vi "Get Item Data.vi"(8 "error in (no error)":errorcluster, 11 "VI":refnum<vi>) -> (0 "error out":errorcluster, 2 "VI Data":T1, 3 "VI out":refnum<vi>)   [LabVIEW 2023, in "VI Properties Editor.lvlib"]
doc: "Gets all item data from the <B>VI</B>."
uses:
  VI Properties Editor.lvlib
  <vilib>/picture/picture.llb/imagedata.ctl
  CTLs/VI Data.ctl
  CTLs/Control Properties.ctl
  CTLs/VI Properties.ctl
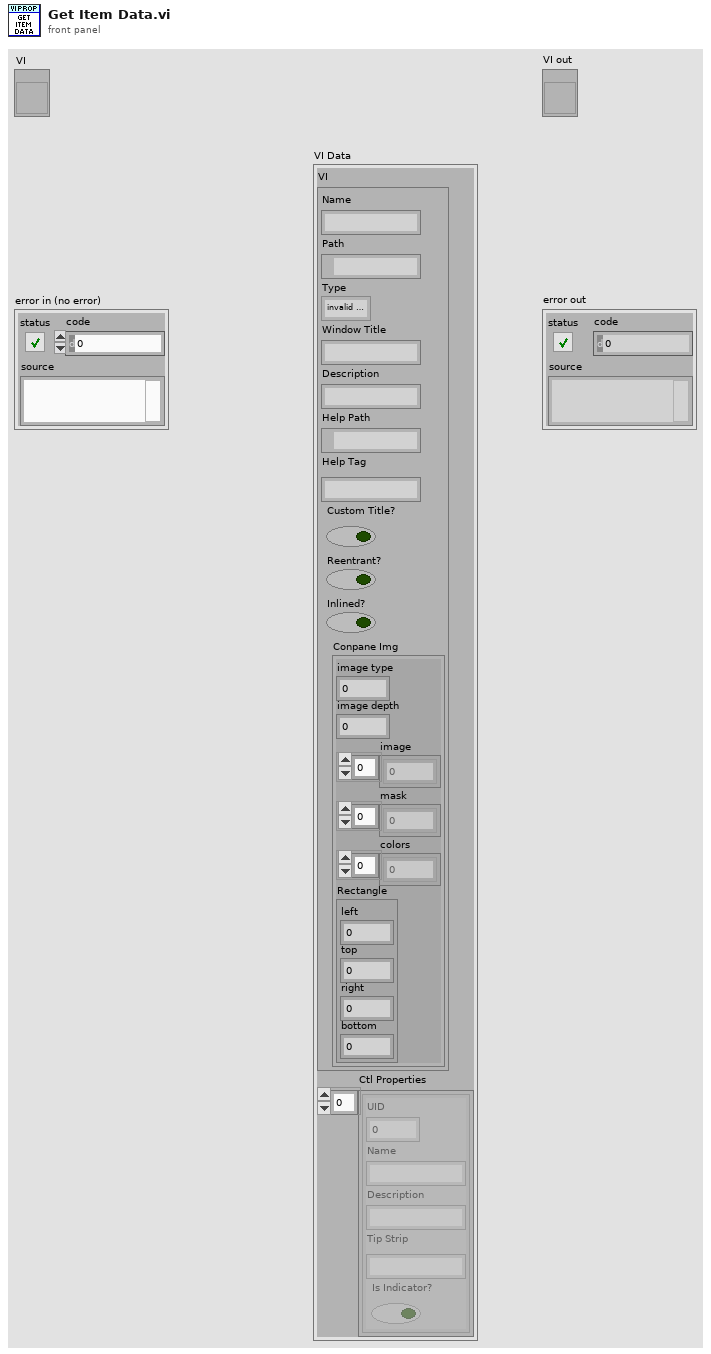
[diagram p1: front panel]
types:
  T1 = typedef "VI Properties Editor.lvlib/VI Data.ctl" = cluster{"VI":T2, "Ctl Properties":T4[]}
  T2 = typedef "VI Properties Editor.lvlib/VI Properties.ctl" = cluster{"Name":string, "Path":path, "Type":enum32{"invalid VI type", "Standard VI", "Control VI", "Global VI", "Polymorphic VI", "Configuration VI", "SubSystem", "Facade VI", "Method VI", "Statechart Diagram VI"}, "Window Title":string, "Description":string, "Help Path":path, "Help Tag":string, "Custom Title?":bool, "Reentrant?":bool, "Inlined?":bool, "Conpane Img":T3}
  T3 = typedef "imagedata.ctl" = cluster{"image type":i32, "image depth":i32, "image":u8[], "mask":u8[], "colors":u32[], "Rectangle":cluster{"left":i16, "top":i16, "right":i16, "bottom":i16}}
  T4 = typedef "VI Properties Editor.lvlib/Control Properties.ctl" = cluster{"UID":i32, "Name":string, "Description":string, "Tip Strip":string, "Is Indicator?":bool}
  T5 = enum32{"invalid VI type", "Standard VI", "Control VI", "Global VI", "Polymorphic VI", "Configuration VI", "SubSystem", "Facade VI", "Method VI", "Statechart Diagram VI"}
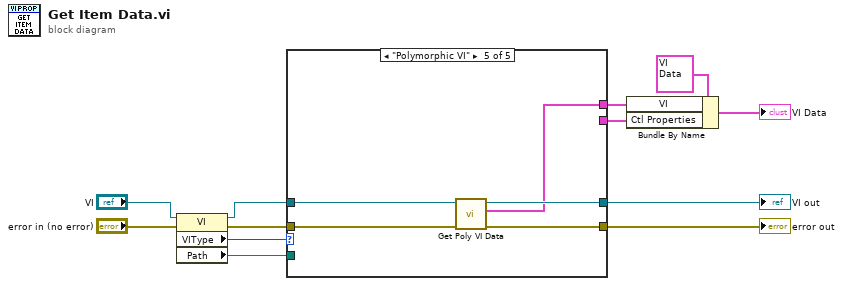
[diagram p0: block diagram]
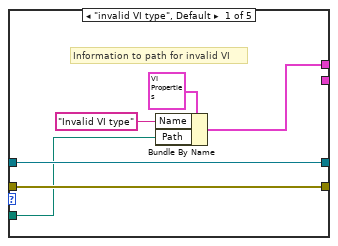
[diagram p2: hidden frame]
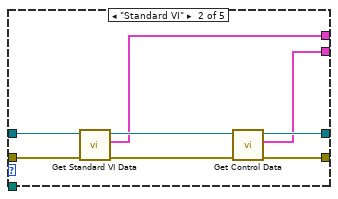
[diagram p3: hidden frame]
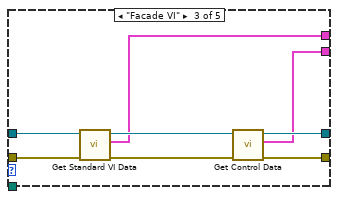
[diagram p4: hidden frame]
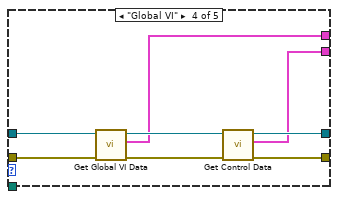
[diagram p5: hidden frame]
diagram:
  n1 = property class="VI"(reference="VI", error in="error in (no error)") -> (reference out=w1:refnum<vi>, error out=w10:errorcluster, "VIType"=w9:T5, "Path"=w4:path)
  n2 = case shown="\"Polymorphic VI\"" w9 {
    tunnel: w10 -> [w18 w24 w32 w42 w43]
    tunnel: w1 -> [w17 w23 w31 w41 w44]
    tunnel: [w14 w20 w28 w35 w45] -> w6
    tunnel: [w18 w21 w29 w37 w47] -> w3
    tunnel: [w17 w25 w33 w38 w46] -> w11
    tunnel: [_ w19 w27 w36 _] -> w7
    tunnel: w4 -> [w13 _ _ _ _]
    frame "invalid VI type", Default {
      # "Information to path for invalid VI"
      n3 = Bundle By Name(cluster=T2 {"Name"="", "Path"=path "", "Type"=enum."invalid VI type", "Window Title"="", "Description"="", "Help Path"=path "", "Help Tag"="", "Custom Title?"=FALSE, "Reentrant?"=FALSE, "Inlined?"=FALSE, "Conpane Img"={"image type"=0, "image depth"=0, "image"=[], "mask"=[], "colors"=[], "Rectangle"={"left"=0, "top"=0, "right"=0, "bottom"=0}}} ("VI Properties"), "Name"="Invalid VI type" ("Help.Tag"), "Path"=w13) -> (w14:T2)
    }
    frame "Standard VI" {
      n4 = call "Get Standard VI Data.vi"("error in (no error)"=w24, "VI in"=w23) -> ("error out"=w22:errorcluster, "VI Properties"=w20:T2, "VI out"=w26:refnum<vi>)  [unwired: 7 in]
      n5 = call "Get Control Data.vi"("error in (no error)"=w22, "VI in"=w26) -> ("error out"=w21:errorcluster, "Control Data"=w19:T4[], "VI out"=w25:refnum<vi>)  [unwired: 7 in]
    }
    frame "Facade VI" {
      n6 = call "Get Standard VI Data.vi"("error in (no error)"=w32, "VI in"=w31) -> ("error out"=w30:errorcluster, "VI Properties"=w28:T2, "VI out"=w34:refnum<vi>)  [unwired: 7 in]
      n7 = call "Get Control Data.vi"("error in (no error)"=w30, "VI in"=w34) -> ("error out"=w29:errorcluster, "Control Data"=w27:T4[], "VI out"=w33:refnum<vi>)  [unwired: 7 in]
    }
    frame "Global VI" {
      n8 = call "Get Global VI Data.vi"("error in (no error)"=w42, "VI in"=w41) -> ("error out"=w40:errorcluster, "VI Properties"=w35:T2, "VI out"=w39:refnum<vi>)  [unwired: 7 in]
      n9 = call "Get Control Data.vi"("error in (no error)"=w40, "VI in"=w39) -> ("error out"=w37:errorcluster, "Control Data"=w36:T4[], "VI out"=w38:refnum<vi>)  [unwired: 7 in]
    }
    frame "Polymorphic VI" {
      n10 = call "Get Poly VI Data.vi"("error in (no error)"=w43, "VI in"=w44) -> ("error out"=w47:errorcluster, "VI Properties"=w45:T2, "VI out"=w46:refnum<vi>)  [unwired: 7 in]
    }
  }
  "error out" <- w3
  "VI out" <- w11
  n11 = Bundle By Name(cluster=T1 {"VI"={"Name"="", "Path"=path "", "Type"=enum."invalid VI type", "Window Title"="", "Description"="", "Help Path"=path "", "Help Tag"="", "Custom Title?"=FALSE, "Reentrant?"=FALSE, "Inlined?"=FALSE, "Conpane Img"={"image type"=0, "image depth"=0, "image"=[], "mask"=[], "colors"=[], "Rectangle"={"left"=0, "top"=0, "right"=0, "bottom"=0}}}, "Ctl Properties"=[]}, "VI"=w6, "Ctl Properties"=w7) -> (→"VI Data":T1)
